vi "parseDataSGL.vi"(8 "error in (no error)":errorcluster, 9 "OverrideSwapBytes":bool, 10 "Index":i32, 11 "U8ArrayParserManualIndexing in":refnum<class "U8ArrayParserManualIndexing.lvclass">) -> (0 "error out":errorcluster, 1 "Data":sgl, 2 "Index out":i32, 3 "U8ArrayParserManualIndexing out":refnum<class "U8ArrayParserManualIndexing.lvclass">)   [LabVIEW 2016, in "RTUtilities.lvlib" / "U8ArrayParserManualIndexing.lvclass"]
uses:
  U8ArrayParserManualIndexing.lvclass
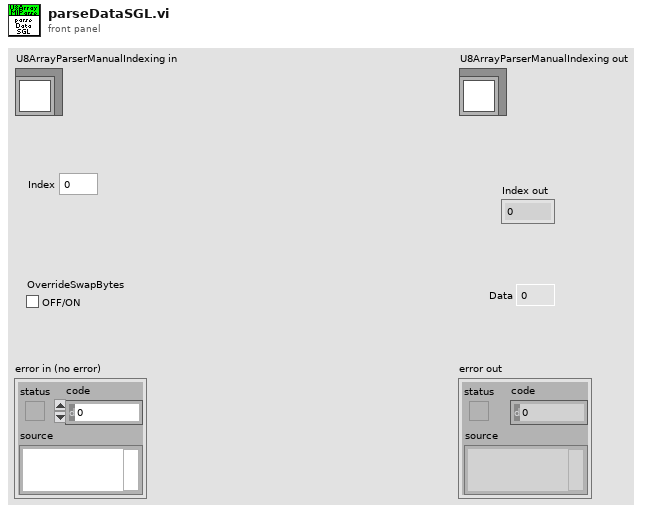
[diagram p1: front panel]
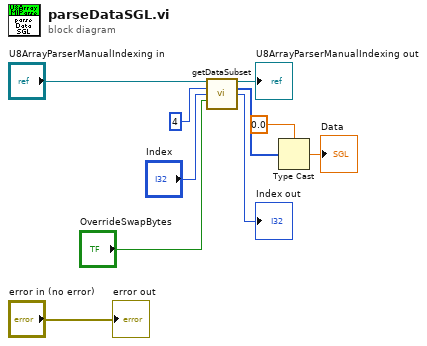
[diagram p0: block diagram]
diagram:
  n1 = call "getDataSubset.vi"("U8ArrayParserManualIndexing in"="U8ArrayParserManualIndexing in", "Length"=4 ("Count"), "Index"="Index", "OverrideSwapBytes"="OverrideSwapBytes") -> ("U8ArrayParserManualIndexing out"=→"U8ArrayParserManualIndexing out":refnum<class "U8ArrayParserManualIndexing.lvclass">, "Data"=w4:u8[], "Index out"=→"Index out":i32)  [unwired: 8 in, 1 out]
  n2 = Type Cast(type=sgl 0.0, x=w4) -> (*(type *) &x=→"Data":sgl)
  "error out" <- "error in (no error)"
